vi "fft_wind_tester_v2.vi"() -> ()   [LabVIEW 2021]
uses:
  <vilib>/measure/NI_MAPro.lvlib
  <vilib>/measure/maspectr.llb/FFT Power Spectrum and PSD for 1 Chan (CDB).vi
panel:
  in  "file path":path
  in  "reciver_params":T1={"min PW"=10, "max PW 2"=30, "max gap"=3, "amplitude bar"=0.0}
  out "Array":T2(array[cluster])
  out "cleanPSD first 4096 sampels":cluster{"f0":dbl, "df":dbl, "magnitude":dbl[]}(graph)
  out "T end":i32[](array[numeric])
  out "F":i32[](graph)
  out "length":u16[](graph)
  out "amp":dbl[](graph)
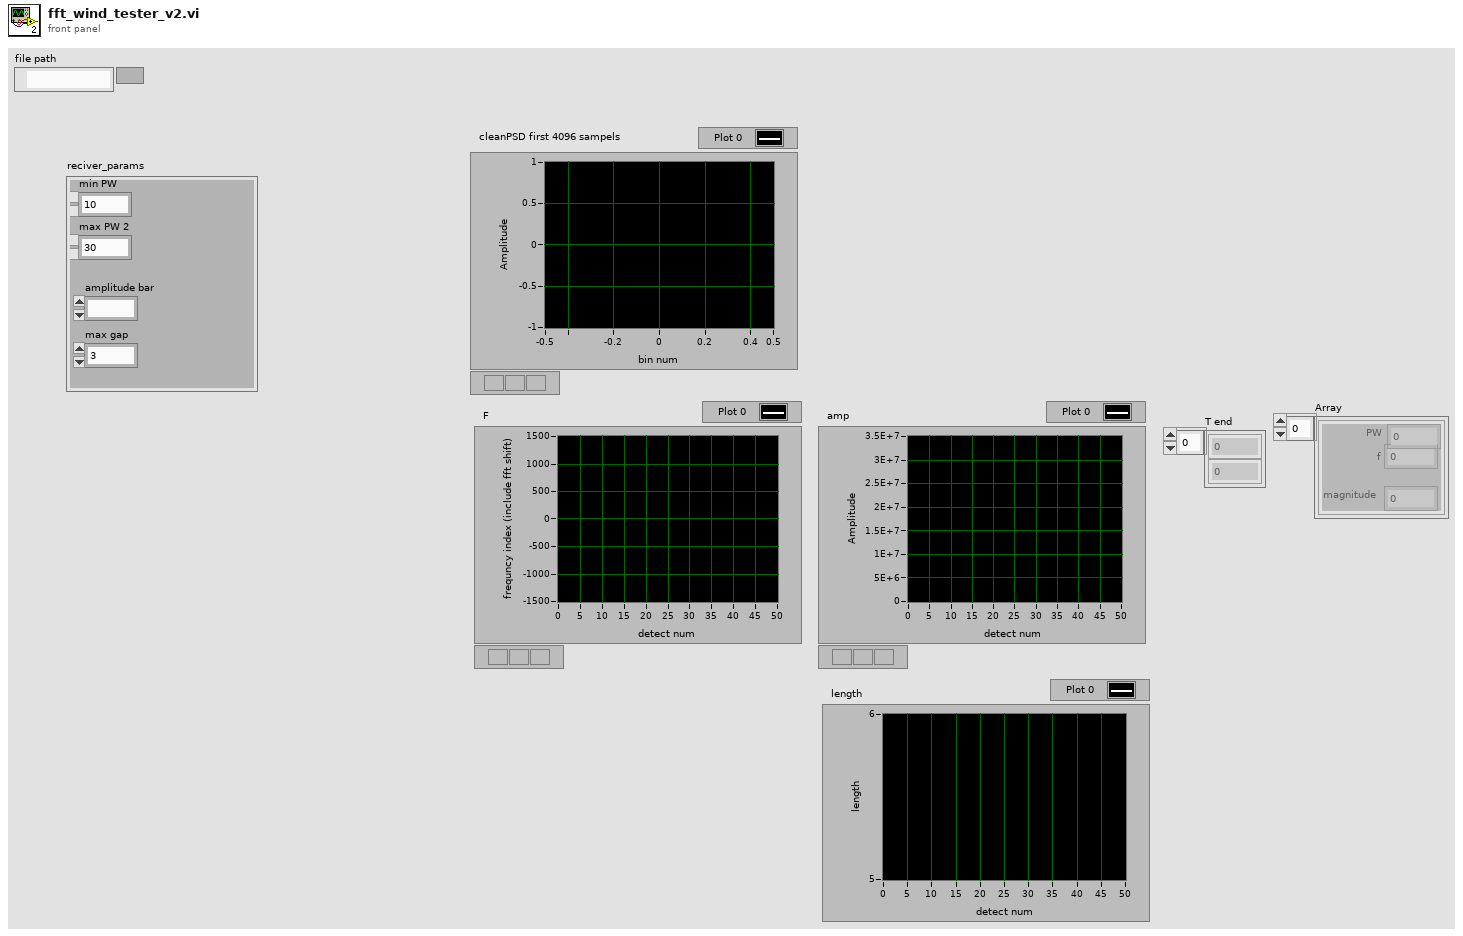
[diagram p1: front panel]
types:
  T1 = cluster{"min PW":u16, "max PW 2":u16, "max gap":u8, "amplitude bar":fxp<+,64,63>}
  T2 = cluster{"PW":u16, "f":i32, "magnitude":fxp<+,32,31>}[]
  T3 = enum16{"open", "open or create", "create or replace", "create", "open (read-only)"}
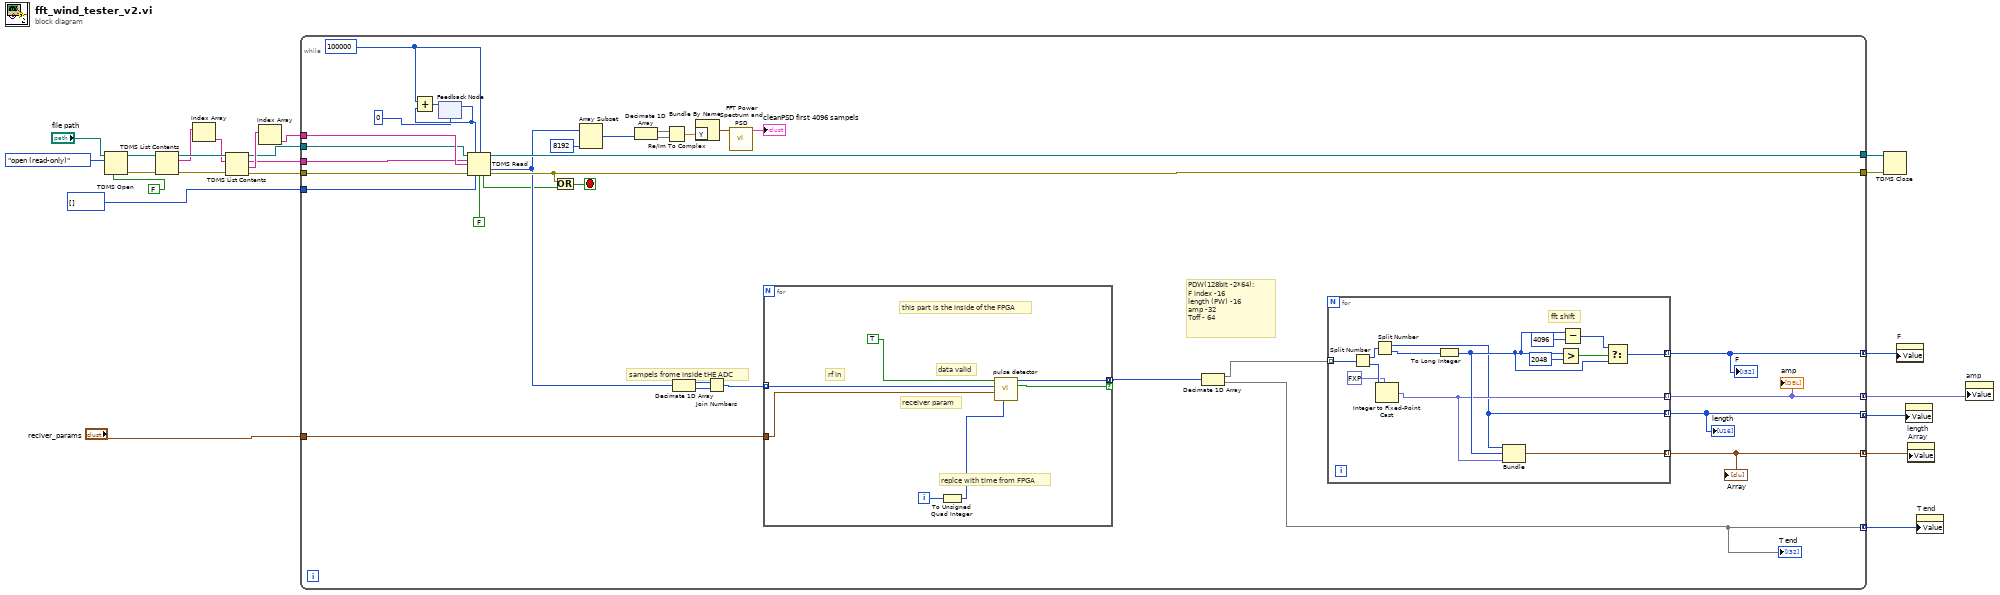
[diagram p0: block diagram]
diagram:
  n1 = TDMS Open(6:FALSE ("disable buffering (T)"), 10:T3."open (read-only)" ("operation"), 11:"file path") -> (0:w15:errorcluster, 3:w20:refnum<k34>)  [unwired: 4 in]
  n2 = TDMS List Contents(4:w15, 7:w20) -> (0:w18:errorcluster, 2:w14:string[], 3:w17:refnum<k34>)  [unwired: 1 in, 1 out]
  n3 = Index Array(array=w14) -> (element=w16:string)  [unwired: 1 in]
  n4 = TDMS List Contents(4:w18, 6:w16, 7:w17) -> (0:w7:errorcluster, 1:w19:string[], 2:w10:string, 3:w9:refnum<k34>)
  n5 = Index Array(array=w19) -> (element=w11:string)  [unwired: 1 in]
  n6 = while {
    tunnel: "reciver_params" -> [w51]
    tunnel: [w48] -> w22
    tunnel: [w31] -> w21
    tunnel: w11 -> [w47]
    tunnel: w10 -> [w46]
    tunnel: w9 -> [w45]
    tunnel: i16[] [] -> [w44]
    tunnel: w7 -> [w38]
    tunnel: [w37] -> w2 mode=concatenating
    tunnel: [w36] -> w3 mode=concatenating
    tunnel: [w35] -> w4 mode=concatenating
    tunnel: [w34] -> w5 mode=concatenating
    tunnel: [w33] -> w6 mode=concatenating
    stop <- w30 stop-if-true
    w50 = i64 100000 ("count (-1: all)")
    # "PDW(128bit -2*64):\nF index -16\nlength (PW) -16\namp -32\nToff - 64"
    # "sampels frome inside tHE ADC"
    n7 = feedback #1(i64 0) -> (w43:i64)
    n8 = Add(x=w50, y=w43) -> (x+y=w49:i64)
    n9 = feedback-in #1(w49) -> ()
    n10 = TDMS Read(0:w45, 1:w43, 2:w50, 5:w46, 7:w47, 11:w38, 12:w44, 13:FALSE ("return channels in file order? (F)")) -> (4:w48:refnum<k34>, 10:w29:i16[], 14:w24:bool, 15:w31:errorcluster)  [unwired: 2 out]
    n11 = Or(x=w31, y=w24) -> (x .or. y?=w30:bool)
    n12 = Array Subset(array=w29, length=8192) -> (w27:i16[])  [unwired: 1 in]
    n13 = Decimate 1D Array(w27) -> (w26:i16[], w25:i16[])
    n14 = Re/Im To Complex(1:w25, 2:w26) -> (0:w54:cdb[])
    n15 = Decimate 1D Array(w29) -> (w53:i16[], w52:i16[])
    n16 = Bundle By Name("Y"=w54) -> (w55:waveform(cdb))  [unwired: 1 in]
    n17 = Join Numbers(hi=w53, lo=w52) -> ((hi.lo)=w28:u32[])
    n18 = call-poly <vilib>:"FFT Power Spectrum and PSD.vi"("time signal"=w55) -> ("Power Spectrum / PSD"=→"cleanPSD first 4096 sampels":cluster{"f0":dbl, "df":dbl, "magnitude":dbl[]})  [unwired: 7 in, 3 out]
    n19 = for {
      tunnel: [w71] -> w40 mode=concatenating if=w74
      tunnel: w28 -> [w76] mode=indexing
      tunnel: w51 -> [w75]
      i -> [w73]
      # "rf in"
      # "receiver param"
      # "data valid"
      # "replce with time from FPGA"
      # "this part is the inside of the FPGA"
      n20 = To Unsigned Quad Integer(1:w73) -> (0:w72:u64)
      n21 = call "pulse detector.vi"("time"=w72, "reciver_params"=w75, "IQ sampels"=w76, "input valid"=TRUE) -> ("output valid"=w74:bool, "data out"=w71:u64[])  [unwired: 6 in]
    }
    n22 = Decimate 1D Array(w40) -> (w39:u64[], w33:u64[])
    "T end" <- w33
    n23 = for {
      tunnel: [w64] -> w37 mode=indexing
      tunnel: [w60] -> w34 mode=indexing
      tunnel: [w59] -> w36 mode=indexing
      tunnel: [w58] -> w35 mode=indexing
      tunnel: w39 -> [w57] mode=indexing
      # "fft shift"
      n24 = Split Number(x=w57) -> (hi(x)=w63:u32, lo(x)=w62:u32)
      n25 = Split Number(x=w63) -> (hi(x)=w58:u16, lo(x)=w69:u16)
      n26 = Integer to Fixed-Point Cast(fixed-point type=fxp<+,32,31> 0.0 ("magnitude"), integer=w62) -> (fixed-point=w59:fxp<+,32,31>)
      n27 = To Long Integer(number=w69) -> (32bit integer=w70:i32)
      n28 = Bundle(w58, w70, "magnitude"=w59) -> (w60:cluster{u16, i32, "magnitude":fxp<+,32,31>})  [unwired: 1 in]
      n29 = Greater?(x=w70, y=u16 2048) -> (0:w66:bool)
      n30 = Subtract(x=w70, y=u16 4096) -> (x-y=w68:i32)
      n31 = Select(t=w68, s=w66, f=w70) -> (s? t:f=w64:i32)
    }
    "length" <- w35
    "F" <- w37
    "amp" <- w36
    "Array" <- w34
  }
  n32 = TDMS Close(8:w21, 11:w22) -> ()  [unwired: 2 out]
  n33 = property on="F" class="WFGraph (strict)"("Value"=w2) -> ()  [unwired: 2 in, 2 out]
  n34 = property on="length" class="WFGraph (strict)"("Value"=w4) -> ()  [unwired: 2 in, 2 out]
  n35 = property on="Array" class="Arr (strict)"("Value"=w5) -> ()  [unwired: 2 in, 2 out]
  n36 = property on="T end" class="Arr (strict)"("Value"=w6) -> ()  [unwired: 2 in, 2 out]
  n37 = property on="amp" class="WFGraph (strict)"("Value"=w3) -> ()  [unwired: 2 in, 2 out]
